vi "Initialize Transfers.vi"(8 "error in (no error)":errorcluster, 11 "transfer group configuration":T1={"name"="", "direction"=enum."Tx", "cycle timing"={"priority"=100, "decimation"=1, "offset"=0}, "thread index"=0, "settings"=[], "transfers"=[], "timeout behavior"=enum."Increment Late Count", "enable buffer conversion"=FALSE} {"transfers"."channels"."string offset" format="%d bytes"}) -> (0 "error out":errorcluster, 2 "max buffer size":u64, 3 "transfer parameters":T10[](array[typedef]))   [LabVIEW 2017, in "UDP.lvlib" / "UDP Transceiver.lvclass"]
uses:
  UDP Transceiver.lvclass
  Transfer Parameters.ctl
  Builds/Data Sharing Framework/Current/Core/DSF Core.lvlibp/Typedefs/DSF Engine Transfer Group Configuration.ctl
  Builds/Data Sharing Framework/Current/Core/DSF Core.lvlibp/Typedefs/DSF Direction.ctl
  Builds/Data Sharing Framework/Current/Core/DSF Core.lvlibp/Typedefs/DSF Timing Info.ctl
  Builds/Data Sharing Framework/Current/Core/DSF Core.lvlibp/Typedefs/DSF Settings Info.ctl
  Builds/Data Sharing Framework/Current/Core/DSF Core.lvlibp/Typedefs/DSF Engine Transfer Configuration.ctl
  Builds/Data Sharing Framework/Current/Core/DSF Core.lvlibp/Typedefs/DSF Byte Order.ctl
  Builds/Data Sharing Framework/Current/Core/DSF Core.lvlibp/Typedefs/DSF Engine Channel Configuration.ctl
  Builds/Data Sharing Framework/Current/Core/DSF Core.lvlibp/Typedefs/DSF Data Type.ctl
  Builds/Data Sharing Framework/Current/Core/DSF Core.lvlibp/Typedefs/DSF Timeout Behavior.ctl
  Builds/Data Sharing Framework/Current/Core/DSF Core.lvlibp/Classes/Configuration/Required Buffer Size (Transfer).vi
  Throw Unknown Setting Error.vi
  Builds/Data Sharing Framework/Current/Core/DSF Core.lvlibp/Classes/Configuration/Configuration Session.lvclass
  Builds/Data Sharing Framework/Current/Core/DSF Core.lvlibp
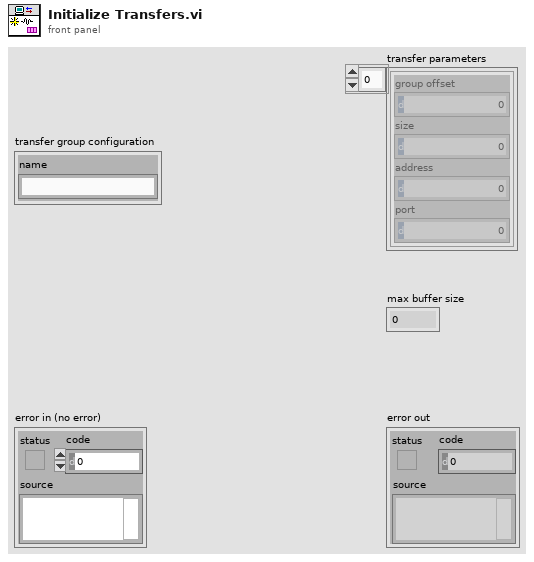
[diagram p1: front panel]
types:
  T1 = typedef "DSF Core.lvlibp/DSF Engine Transfer Group Configuration.ctl" = cluster{"name":string, "direction":T2, "cycle timing":T3, "thread index":u8, "settings":T4, "transfers":T5[], "timeout behavior":T9, "enable buffer conversion":bool}
  T2 = typedef "DSF Core.lvlibp/DSF Direction.ctl" = enum8{"Tx", "Rx"}
  T3 = typedef "DSF Core.lvlibp/DSF Timing Info.ctl" = cluster{"priority":u64, "decimation":u64, "offset":u64}
  T4 = typedef "DSF Core.lvlibp/DSF Settings Info.ctl" = cluster{"component":string, "name":string, "values":cluster{"key":string, "value":string}[]}[]
  T5 = typedef "DSF Core.lvlibp/DSF Engine Transfer Configuration.ctl" = cluster{"name":string, "byte order":T6, "settings":T4, "channels":T7[]}
  T6 = typedef "DSF Core.lvlibp/DSF Byte Order.ctl" = enum8{"big-endian", "little-endian"}
  T7 = typedef "DSF Core.lvlibp/DSF Engine Channel Configuration.ctl" = cluster{"string offset":u64, "name":string, "units":string, "engine data type":T8, "string data type":T8, "settings":T4}
  T8 = typedef "DSF Core.lvlibp/DSF Data Type.ctl" = enum8{"Bool", "SGL", "DBL", "I8", "I16", "I32", "I64", "U8", "U16", "U32", "U64"}
  T9 = typedef "DSF Core.lvlibp/DSF Timeout Behavior.ctl" = enum8{"Increment Late Count", "Throw Error"}
  T10 = typedef "UDP.lvlib/UDP Transceiver.lvclass/Transfer Parameters.ctl" = cluster{"group offset":u64, "size":u64, "address":u32, "port":u16}
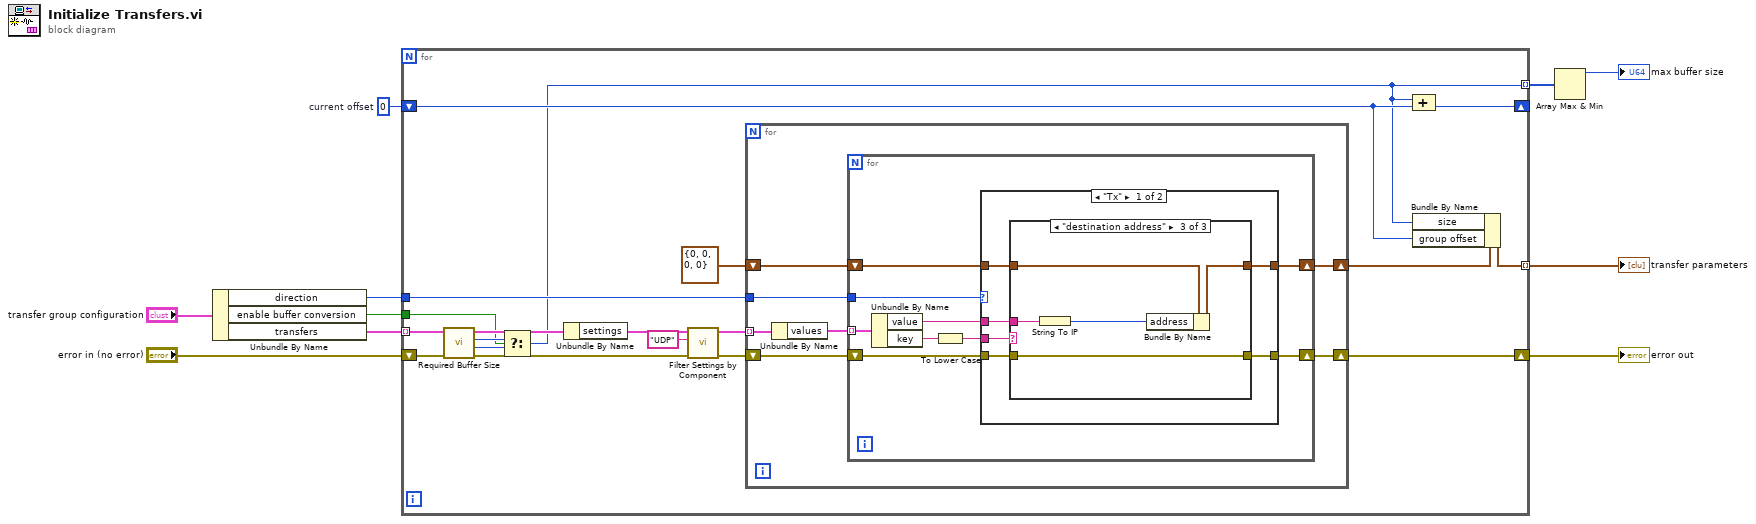
[diagram p0: block diagram]
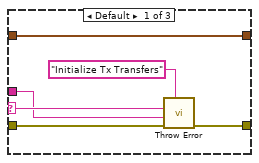
[diagram p2: hidden frame]
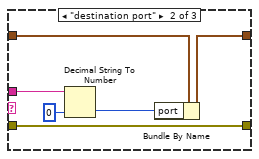
[diagram p3: hidden frame]
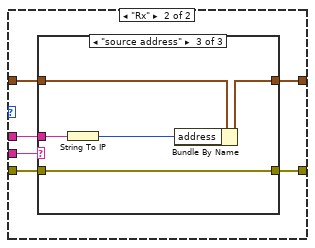
[diagram p4: hidden frame]
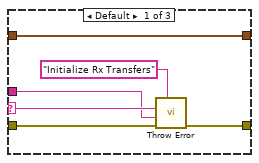
[diagram p5: hidden frame]
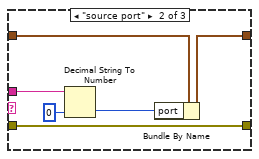
[diagram p6: hidden frame]
diagram:
  w1 = u64 0  # current offset
  n1 = Unbundle By Name("transfer group configuration") -> ("direction"=w2:T2, "enable buffer conversion"=w3:bool, "transfers"=w4:T5[])
  n2 = for {
    shift-right: [w29] -> w8
    shift-left: "error in (no error)" -> [w27]
    tunnel: w4 -> [w28] mode=indexing
    tunnel: [w11] -> w9 mode=indexing
    tunnel: [w13] -> w7 mode=indexing
    tunnel: w3 -> [w16]
    tunnel: w2 -> [w18]
    shift-right: [w15] -> _
    shift-left: w1 -> [w14]
    n3 = call-poly "Required Buffer Size.vi"("error in (no error)"=w27, "Transfer Configuration in"=w28) -> ("error out"=w25:errorcluster, "engine buffer size"=w17:u64, "string buffer size"=w20:u64, "Transfer Configuration out"=w26:T5)  [unwired: 6 in]
    n4 = Select(t=w20, s=w16, f=w17) -> (s? t:f=w13:u64)
    n5 = Unbundle By Name(w26) -> ("settings"=w21:T4)
    n6 = call "Filter Settings by Component.vi"("error in (no error)"=w25, "component"="UDP", "settings"=w21) -> ("error out"=w24:errorcluster, "filtered settings"=w22:T4)  [unwired: 7 in]
    n7 = for {
      tunnel: w22 -> [w32] mode=indexing
      shift-right: [w34] -> w12
      shift-left: T10 {"group offset"=0, "size"=0, "address"=0, "port"=0} ("Transfer Tx") -> [w35]
      shift-right: [w36] -> w29
      shift-left: w24 -> [w33]
      tunnel: w18 -> [w30]
      n8 = Unbundle By Name(w32) -> ("values"=w31:cluster{"key":string, "value":string}[])
      n9 = for {
        tunnel: w31 -> [w45] mode=indexing
        shift-right: [w40] -> w36
        shift-left: w33 -> [w44]
        shift-right: [w42] -> w34
        shift-left: w35 -> [w43]
        tunnel: w30 -> [w37]
        n10 = Unbundle By Name(w45) -> ("value"=w41:string, "key"=w39:string)
        n11 = To Lower Case(string=w39) -> (all lower case string=w38:string)
        n12 = case shown="\"Tx\"" w37 {
          tunnel: w44 -> [w51 w74]
          tunnel: w43 -> [w50 w71]
          tunnel: [w49 w70] -> w42
          tunnel: w41 -> [w48 w72]
          tunnel: [w47 w69] -> w40
          tunnel: w38 -> [w46 w73]
          frame "Tx" {
            n13 = case shown="\"destination address\"" w46 {
              selector: w46 -> [w53 _ _]
              tunnel: w48 -> [w52 w63 w67]
              tunnel: w51 -> [w55 w60 w68]
              tunnel: [w54 w60 w68] -> w47
              tunnel: w50 -> [w57 w59 w64]
              tunnel: [w57 w58 w65] -> w49
              frame Default {
                n14 = call-poly "Throw Error.vi"("source vi name"="Initialize Tx Transfers", "error in (no error)"=w55, "value"=w52, "key"=w53) -> ("error out"=w54:errorcluster)  [unwired: 7 in]
              }
              frame "destination port" {
                n15 = Decimal String To Number(string=w63, default (0L)=u16 0 ("default (0 I32)")) -> (number=w61:u16)  [unwired: 1 in, 1 out]
                n16 = Bundle By Name(cluster=w59, "port"=w61) -> (w58:T10)
              }
              frame "destination address" {
                n17 = String To IP(1:w67) -> (0:w66:u32)
                n18 = Bundle By Name(cluster=w64, "address"=w66) -> (w65:T10)
              }
            }
          }
          frame "Rx" {
            n19 = case shown="\"source address\"" w73 {
              selector: w73 -> [w76 _ _]
              tunnel: w72 -> [w75 w86 w88]
              tunnel: w74 -> [w79 w83 w91]
              tunnel: [w78 w83 w91] -> w69
              tunnel: w71 -> [w77 w82 w90]
              tunnel: [w77 w81 w89] -> w70
              frame Default {
                n20 = call-poly "Throw Error.vi"("source vi name"="Initialize Rx Transfers", "error in (no error)"=w79, "value"=w75, "key"=w76) -> ("error out"=w78:errorcluster)  [unwired: 7 in]
              }
              frame "source port" {
                n21 = Decimal String To Number(string=w86, default (0L)=u16 0 ("default (0 I32)")) -> (number=w84:u16)  [unwired: 1 in, 1 out]
                n22 = Bundle By Name(cluster=w82, "port"=w84) -> (w81:T10)
              }
              frame "source address" {
                n23 = String To IP(1:w88) -> (0:w87:u32)
                n24 = Bundle By Name(cluster=w90, "address"=w87) -> (w89:T10)
              }
            }
          }
        }
      }
    }
    n25 = Compound Arithmetic op=ADD(w13, w14) -> (w15:u64)
    n26 = Bundle By Name(cluster=w12, "size"=w13, "group offset"=w14) -> (w11:T10)
  }
  "error out" <- w8
  "transfer parameters" <- w9
  n27 = Array Max & Min(array=w7) -> (max value=→"max buffer size":u64)  [unwired: 3 out]
